vi "ALTS-2015 Write Result to DB.vi"(7 "Options":T1, 8 "Error In":errorcluster, 11 "Command reference In":T2) -> (0 "Error Out":errorcluster, 3 "Command reference Out":T2)   [LabVIEW 2013]
uses:
  <vilib>/addons/database/Command.llb/Cmd ObjectReference.ctl
  Controls/ALTS-2015 write DB Result cases.ctl
  <vilib>/addons/database/Command.llb/Cmd Set Parameter Value (C).vi
  <vilib>/addons/database/Command.llb/Cmd Execute.vi
  <vilib>/addons/database/Recordset.llb/Rec Destroy - Command.vi
  <vilib>/addons/database/NI_Database_API.lvlib
panel:
  in  "Value":string="1500"
  in  "Parameter Value ID":i32=229
  in  "Serial Number":string="070125ACC0018"
  in  "TEST STAND ID":i32=1 format="%0#4_1f"
  in  "USER ID":string="ENGINEER"
  in  "DATE":string="20070423124522"
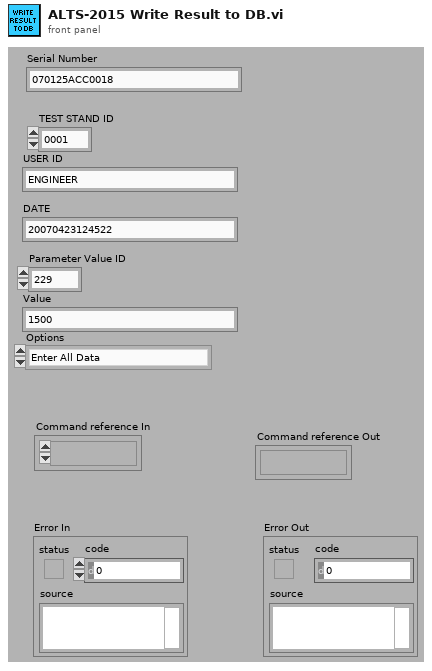
[diagram p1: front panel]
types:
  T1 = typedef "ALTS-2015 write DB Result cases.ctl" = enum16{"Enter All Data", "Enter WO & SN"}
  T2 = typedef "NI_Database_API.lvlib/Cmd ObjectReference.ctl" = refnum<k1>
  T3 = typedef "ALTS-2015 DB Result Cluster.ctl" = cluster{"Sensor_Name":string, "SN":string, "Work_order_Number":string, "User1":string, "User2":string, "User3":string, "User4":string, "Pressure":dbl, "Flow":dbl, "Test_Result":string, "Test_Time":string, "Repair Code":string}
  T4 = typedef "NI_Database_API.lvlib/Cmd-Rec Object Reference.ctl" = refnum<k1>
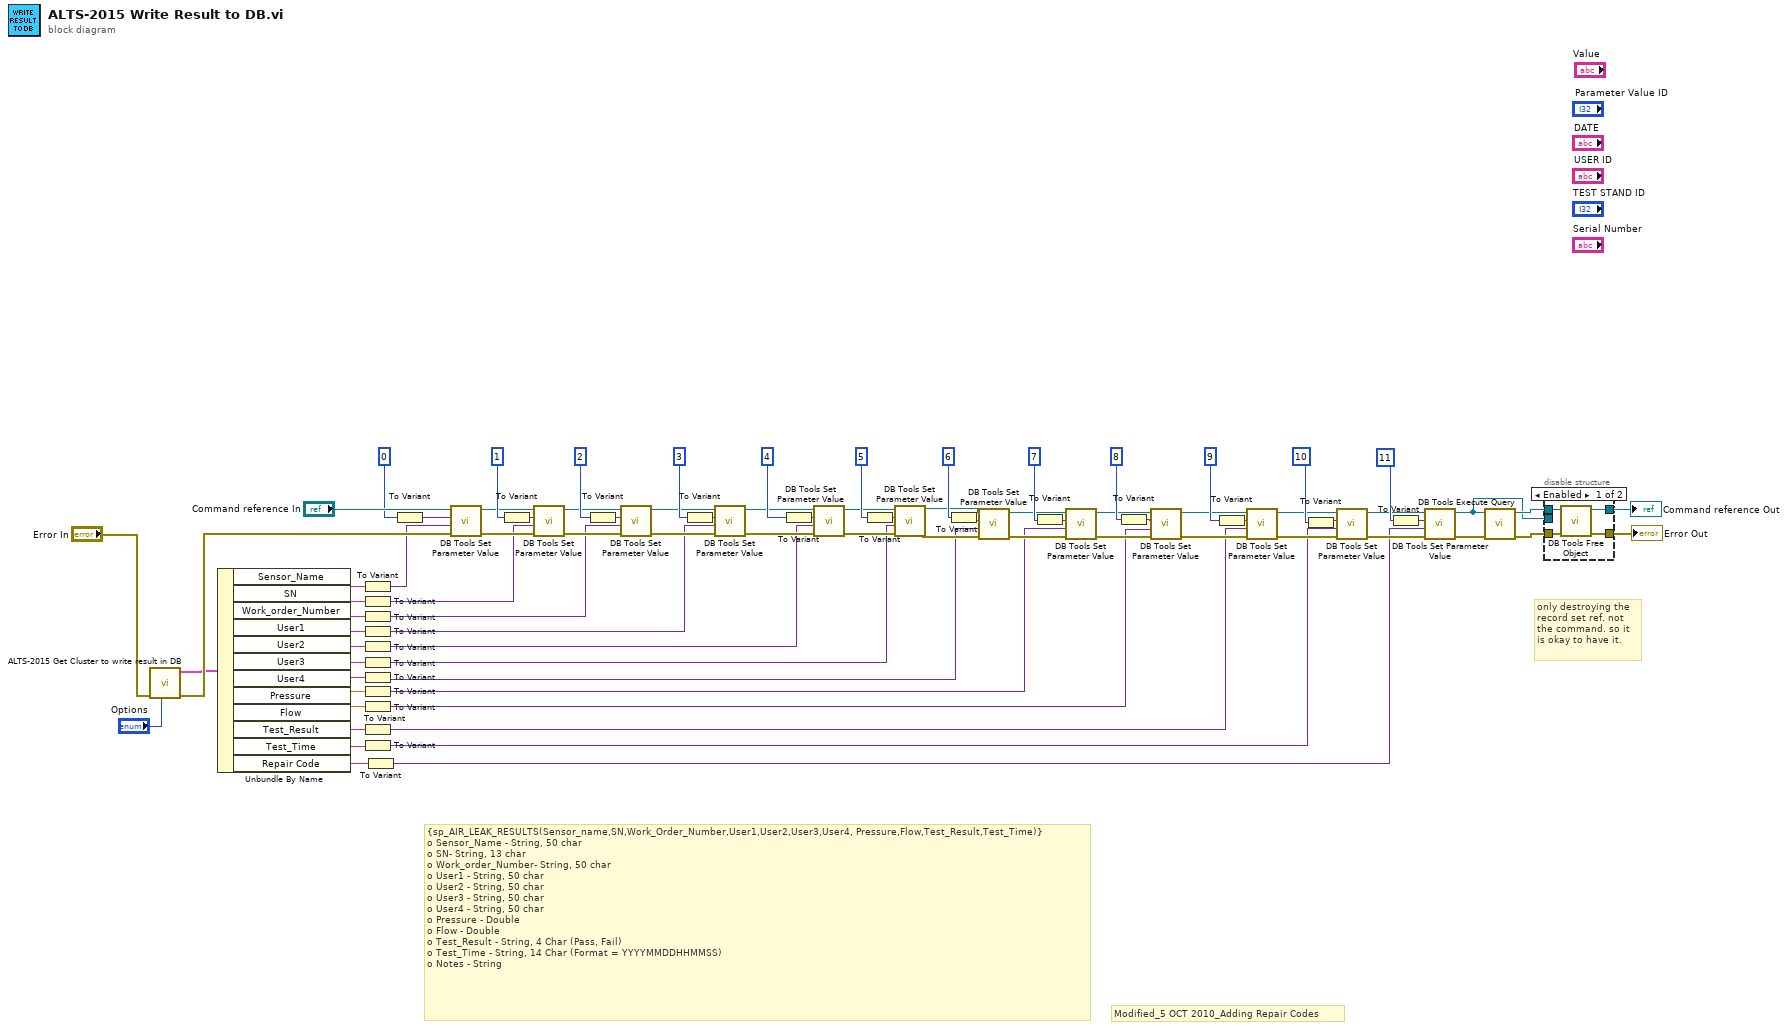
[diagram p0: block diagram]
diagram:
  # "Modified_5 OCT 2010_Adding Repair Codes"
  # "only destroying the\nrecord set ref. not \nthe command. so it\nis okay to have it."
  # "{sp_AIR_LEAK_RESULTS(Sensor_name,SN,Work_Order_Number,User1,User2,User3,User4, Pressure,Flow,Test_Result,Test_Time)}\no\tSensor_Name - String, 50 char\no\tSN- String, 13 char\no\tWork_order_Number- String, 50 char\no\tUser1 - String, 50 char\no\tUser2 - String, 50 char\no\tUser3 - String, 50 char\no\tUser4 - String, 50 char\no\tPressure - Double\no\tFlow - Double\no\tTest_Result - String, 4 Char (Pass, Fail)\no\tTest_Time - String, 14 Char (Format = YYYYMMDDHHMMSS)\no\tNotes - String"
  n1 = call "ALTS-2015 Get Cluster to write result in DB.vi"("Options"="Options", "error in"="Error In") -> ("error out"=w81:errorcluster, "DB Result Cluster Out"=w21:T3)  [unwired: 8 in]
  n2 = Unbundle By Name(w21) -> ("Sensor_Name"=w20:string, "SN"=w19:string, "Work_order_Number"=w18:string, "User1"=w17:string, "User2"=w16:string, "User3"=w15:string, "User4"=w14:string, "Pressure"=w13:dbl, "Flow"=w12:dbl, "Test_Result"=w11:string, "Test_Time"=w10:string, "Repair Code"=w3:string)
  n3 = To Variant(anything=w20) -> (Variant=w59:variant)
  n4 = To Variant(anything=w19) -> (Variant=w60:variant)
  n5 = To Variant(anything=w18) -> (Variant=w32:variant)
  n6 = To Variant(anything=w17) -> (Variant=w31:variant)
  n7 = To Variant(anything=w16) -> (Variant=w30:variant)
  n8 = To Variant(anything=w15) -> (Variant=w29:variant)
  n9 = To Variant(anything=w14) -> (Variant=w28:variant)
  n10 = To Variant(anything=w13) -> (Variant=w27:variant)
  n11 = To Variant(anything=w12) -> (Variant=w26:variant)
  n12 = To Variant(anything=w11) -> (Variant=w25:variant)
  n13 = To Variant(anything=w10) -> (Variant=w23:variant)
  n14 = To Variant(anything=w3) -> (Variant=w2:variant)
  n15 = To Variant(anything=0 ("TEST STAND ID")) -> (Variant=w58:variant)
  n16 = call-poly <vilib>:"DB Tools Set Parameter Value.vi"("error in (no error)"=w81, "value"=w59, "parameter index"=w58, "command reference"="Command reference In") -> ("error out"=w66:errorcluster, "command reference out"=w65:T2)  [unwired: 4 in]
  n17 = To Variant(anything=1 ("TEST STAND ID")) -> (Variant=w57:variant)
  n18 = call-poly <vilib>:"DB Tools Set Parameter Value.vi"("error in (no error)"=w66, "value"=w60, "parameter index"=w57, "command reference"=w65) -> ("error out"=w53:errorcluster, "command reference out"=w54:T2)  [unwired: 4 in]
  n19 = To Variant(anything=2 ("TEST STAND ID")) -> (Variant=w56:variant)
  n20 = call-poly <vilib>:"DB Tools Set Parameter Value.vi"("error in (no error)"=w53, "value"=w32, "parameter index"=w56, "command reference"=w54) -> ("error out"=w63:errorcluster, "command reference out"=w64:T2)  [unwired: 4 in]
  n21 = To Variant(anything=3 ("TEST STAND ID")) -> (Variant=w55:variant)
  n22 = call-poly <vilib>:"DB Tools Set Parameter Value.vi"("error in (no error)"=w63, "value"=w31, "parameter index"=w55, "command reference"=w64) -> ("error out"=w33:errorcluster, "command reference out"=w34:T2)  [unwired: 4 in]
  n23 = To Variant(anything=4 ("TEST STAND ID")) -> (Variant=w46:variant)
  n24 = call-poly <vilib>:"DB Tools Set Parameter Value.vi"("error in (no error)"=w33, "value"=w30, "parameter index"=w46, "command reference"=w34) -> ("error out"=w44:errorcluster, "command reference out"=w43:T2)  [unwired: 4 in]
  n25 = To Variant(anything=5 ("TEST STAND ID")) -> (Variant=w52:variant)
  n26 = call-poly <vilib>:"DB Tools Set Parameter Value.vi"("error in (no error)"=w44, "value"=w29, "parameter index"=w52, "command reference"=w43) -> ("error out"=w41:errorcluster, "command reference out"=w42:T2)  [unwired: 4 in]
  n27 = To Variant(anything=6 ("TEST STAND ID")) -> (Variant=w45:variant)
  n28 = call-poly <vilib>:"DB Tools Set Parameter Value.vi"("error in (no error)"=w41, "value"=w28, "parameter index"=w45, "command reference"=w42) -> ("error out"=w40:errorcluster, "command reference out"=w37:T2)  [unwired: 4 in]
  n29 = To Variant(anything=7 ("TEST STAND ID")) -> (Variant=w51:variant)
  n30 = call-poly <vilib>:"DB Tools Set Parameter Value.vi"("error in (no error)"=w40, "value"=w27, "parameter index"=w51, "command reference"=w37) -> ("error out"=w39:errorcluster, "command reference out"=w36:T2)  [unwired: 4 in]
  n31 = To Variant(anything=8 ("TEST STAND ID")) -> (Variant=w50:variant)
  n32 = call-poly <vilib>:"DB Tools Set Parameter Value.vi"("error in (no error)"=w39, "value"=w26, "parameter index"=w50, "command reference"=w36) -> ("error out"=w38:errorcluster, "command reference out"=w35:T2)  [unwired: 4 in]
  n33 = To Variant(anything=9 ("TEST STAND ID")) -> (Variant=w49:variant)
  n34 = call-poly <vilib>:"DB Tools Set Parameter Value.vi"("error in (no error)"=w38, "value"=w25, "parameter index"=w49, "command reference"=w35) -> ("error out"=w48:errorcluster, "command reference out"=w47:T2)  [unwired: 4 in]
  n35 = To Variant(anything=10 ("TEST STAND ID")) -> (Variant=w24:variant)
  n36 = call-poly <vilib>:"DB Tools Set Parameter Value.vi"("error in (no error)"=w48, "value"=w23, "parameter index"=w24, "command reference"=w47) -> ("error out"=w5:errorcluster, "command reference out"=w7:T2)  [unwired: 4 in]
  n37 = To Variant(anything=11 ("TEST STAND ID")) -> (Variant=w9:variant)
  n38 = call-poly <vilib>:"DB Tools Set Parameter Value.vi"("error in (no error)"=w5, "value"=w2, "parameter index"=w9, "command reference"=w7) -> ("error out"=w4:errorcluster, "command reference out"=w6:T2)  [unwired: 4 in]
  n39 = call-poly <vilib>:"DB Tools Execute Query.vi"("error in (no error)"=w4, "command reference"=w6) -> ("error out"=w62:errorcluster, "command-recordset reference"=w61:T4)  [unwired: 6 in]
  n40 = disable-structure shown="Enabled" {
    disable-tunnel: [w85 w87] -> w78
    disable-tunnel: w62 -> [w84 w87]
    disable-tunnel: w61 -> [w83 _]
    disable-tunnel: [w82 w86] -> w80
    disable-tunnel: w6 -> [_ w86]
    frame Enabled {
      n41 = call-poly <vilib>:"DB Tools Free Object.vi"("error in (no error)"=w84, "command-recordset reference"=w83) -> ("error out"=w85:errorcluster, "command reference"=w82:T2)  [unwired: 8 in]
    }
    frame Disabled {
    }
  }
  "Error Out" <- w78
  "Command reference Out" <- w80
